vi "ORS_PeakHoldComputeGraph.vi"(8 "new data":dbl[](array[numeric]), 11 "graph array in":dbl[][](array[numeric])) -> (3 "graph array out":dbl[][](array[numeric]))   [LabVIEW 2014]
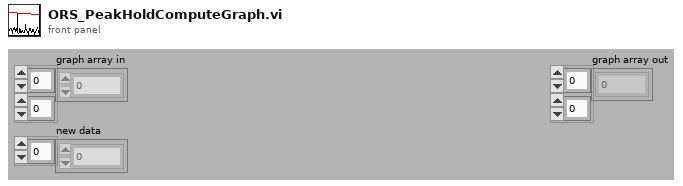
[diagram p1: front panel]
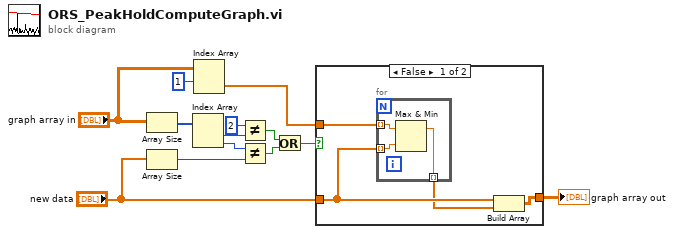
[diagram p0: block diagram]
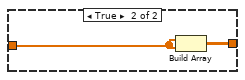
[diagram p2: hidden frame]
diagram:
  n1 = Array Size(array="graph array in") -> (size(s)=w12:i32[])
  n2 = Array Size(array="new data") -> (size(s)=w8:i32)
  n3 = Index Array(array=w12) -> (element #1=w11:i32, element #2=w9:i32)  [unwired: 2 in]
  n4 = Index Array(array="graph array in", index (row)=1) -> (element=w1:dbl[])  [unwired: 1 in]
  n5 = Not Equal?(x=2, y=w11) -> (x != y?=w6:bool)
  n6 = Not Equal?(x=w9, y=w8) -> (x != y?=w7:bool)
  n7 = Or(x=w6, y=w7) -> (x .or. y?=w5:bool)
  n8 = case shown="False" w5 {
    tunnel: "new data" -> [w16 w22]
    tunnel: [w17 w21] -> w3
    tunnel: w1 -> [w15 _]
    frame False {
      n9 = for {
        tunnel: w16 -> [w19] mode=indexing
        tunnel: w15 -> [w20] mode=indexing
        tunnel: [w18] -> w14 mode=indexing
        n10 = Max & Min(x=w20, y=w19) -> (max(x,y)=w18:dbl)  [unwired: 1 out]
      }
      n11 = Build Array(w16, w14) -> (w17:dbl[][])
    }
    frame True {
      n12 = Build Array(w22, w22) -> (w21:dbl[][])
    }
  }
  "graph array out" <- w3
